vi "FT_Read_FT2232H_EEPROM.vi"(0 "Handle":u32) -> (1 "FT_Status":u32(ring) items=["FT_OK", "FT_INVALID_HANDLE", "FT_DEVICE_NOT_FOUND", "FT_DEVICE_NOT_OPENED", "FT_IO_ERROR", "FT_INSUFFICIENT_RESOURCES", "FT_INVALID_PARAMETER", "FT_INVALID_BAUD_RATE", "FT_DEVICE_NOT_OPENED_FOR_ERASE", "FT_DEVICE_NOT_OPENED_FOR_WRITE", "FT_FAILED_TO_WRITE_DEVICE", "FT_EEPROM_READ_FAILED", "FT_EEPROM_WRITE_FAILED", "FT_EEPROM_ERASE_FAILED", "FT_EEPROM_NOT_PRESENT", "FT_EEPROM_NOT_PROGRAMMED", "FT_INVALID_ARGS", "FT_NOT_SUPPORTED", "FT_OTHER_ERROR"], 2 "FT2232H EEPROM Contents":T1={"Vendor ID"=0, "Product ID"=0, "Manufacturer"="", "Manufacturer ID"="", "Description"="", "Serial Number"="", "Max Power (mA)"=0, "PnP"=0, "Self Powered"=0, "Remote Wake-Up"=0, "Pull Down Enable"=0, "Serial Number Enable 7"=0, "AL Slow Slew"=0, "AL Schmitt Input"=0, "AL Drive Current"=4, "AH Slow Slew"=0, "AH Schmitt Input"=0, "AH Drive Current"=4, "BL Slow Slew"=0, "BL Schmitt Input"=0, "BL Drive Current"=4, "BH Slow Slew"=0, "BH Schmitt Input"=0, "BH Drive Current"=4, "A Is 245 FIFO"=0, "A Is CPU FIFO"=0, "A Is Fast Serial"=0, "A Is VCP"=0, "B Is 245 FIFO"=0, "B Is CPU FIFO"=0, "B Is Fast Serial"=0, "B Is VCP"=0, "Power Save"=0} {"Power Save" items=["Disabled", "Enabled"]; "B Is VCP" items=["D2XX", "VCP"]; "B Is Fast Serial" items=["Disabled", "Enabled"]; "B Is CPU FIFO" items=["Disabled", "Enabled"]; "B Is 245 FIFO" items=["UART", "FIFO"]; "A Is VCP" items=["D2XX", "VCP"]; "A Is Fast Serial" items=["Disabled", "Enabled"]; "A Is CPU FIFO" items=["Disabled", "Enabled"]; "A Is 245 FIFO" items=["UART", "FIFO"]; "BH Drive Current" items=["4mA"=4, "8mA"=8, "12mA"=12, "16mA"=16]; "BH Schmitt Input" items=["Disabled", "Enabled"]; "BH Slow Slew" items=["Disabled", "Enabled"]; "BL Drive Current" items=["4mA"=4, "8mA"=8, "12mA"=12, "16mA"=16]; "BL Schmitt Input" items=["Disabled", "Enabled"]; "BL Slow Slew" items=["Disabled", "Enabled"]; "AH Drive Current" items=["4mA"=4, "8mA"=8, "12mA"=12, "16mA"=16]; "AH Schmitt Input" items=["Disabled", "Enabled"]; "AH Slow Slew" items=["Disabled", "Enabled"]; "AL Drive Current" items=["4mA"=4, "8mA"=8, "12mA"=12, "16mA"=16]; "AL Schmitt Input" items=["Disabled", "Enabled"]; "AL Slow Slew" items=["Disabled", "Enabled"]; "Serial Number Enable 7" items=["Disabled", "Enabled"]; "Pull Down Enable" items=["Disabled", "Enabled"]; "Remote Wake-Up" items=["Disabled", "Enabled"]; "Self Powered" items=["Bus Powered", "Self Powered"]; "PnP" items=["Disabled", "Enabled"]})   [LabVIEW 2019, in "D2XX_Functions.lvlib"]
uses:
  <userlib>/LevyLab/Relay Box/D2XX_Functions/D2XX_Functions.lvlib
  <userlib>/LevyLab/Relay Box/D2XX_Functions/i386/ftd2xx.dll
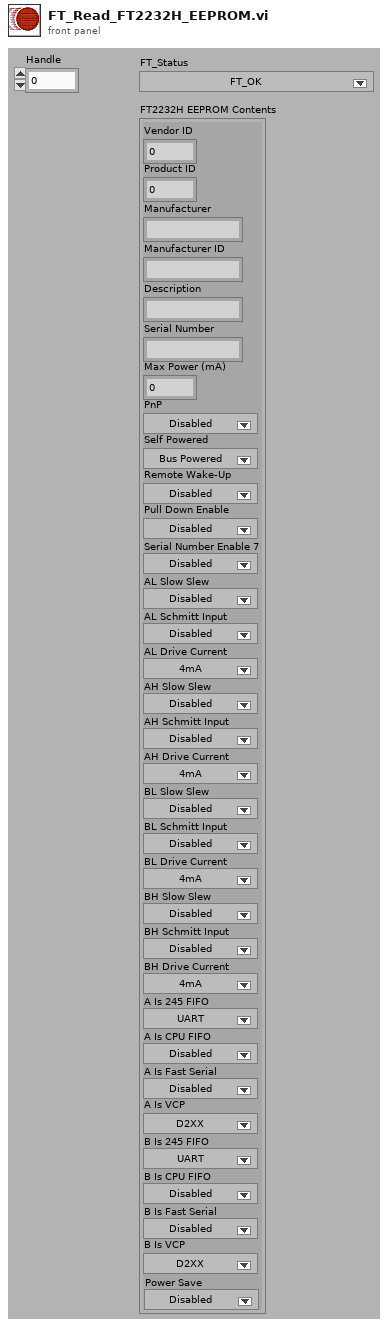
[diagram p1: front panel]
types:
  T1 = cluster{"Vendor ID":u16, "Product ID":u16, "Manufacturer":string, "Manufacturer ID":string, "Description":string, "Serial Number":string, "Max Power (mA)":u16, "PnP":u16, "Self Powered":u16, "Remote Wake-Up":u16, "Pull Down Enable":u8, "Serial Number Enable 7":u8, "AL Slow Slew":u8, "AL Schmitt Input":u8, "AL Drive Current":u8, "AH Slow Slew":u8, "AH Schmitt Input":u8, "AH Drive Current":u8, "BL Slow Slew":u8, "BL Schmitt Input":u8, "BL Drive Current":u8, "BH Slow Slew":u8, "BH Schmitt Input":u8, "BH Drive Current":u8, "A Is 245 FIFO":u8, "A Is CPU FIFO":u8, "A Is Fast Serial":u8, "A Is VCP":u8, "B Is 245 FIFO":u8, "B Is CPU FIFO":u8, "B Is Fast Serial":u8, "B Is VCP":u8, "Power Save":u8}
  T2 = cluster{"Signature 1":u32, "Signature 2":u32, "Version":u32, "Vendor ID":u16, "Product ID":u16, "Manufacturer":u32, "Manufacturer ID":u32, "Description":u32, "Serial Number":u32, "Max Power (mA)":u16, "PnP":u16, "Self Powered":u16, "Remote Wake-Up":u16, "Rev4":u8, "Iso In":u8, "Iso Out":u8, "Pull Down Enable":u8, "Serial Number Enable":u8, "USB Version Enable":u8, "USB Version":u16, "Rev5":u8, "Iso In A":u8, "Iso In B":u8, "Iso Out A":u8, "Iso Out B":u8, "Pull Down Enable 5":u8, "Serial Number Enable 5":u8, "USB Version Enable 5":u8, "USB Version 5":u16, "A Is High Current":u8, "B Is High Current":u8, "A Is 245 FIFO":u8, "A Is CPU FIFO":u8, "A Is Fast Serial":u8, "A Is VCP":u8, "B Is 245 FIFO":u8, "B Is CPU FIFO":u8, "B Is Fast Serial":u8, "B Is VCP":u8, "Use Ext Osc":u8, "High Drive IOs":u8, "Endpoint Size":u8, "Pull Down Enable R":u8, "Serial Number Enable R":u8, "Invert TXD":u8, "Invert RXD":u8, "Invert RTS":u8, "Invert CTS":u8, "Invert DTR":u8, "Invert DSR":u8, "Invert DCD":u8, "Invert RI":u8, "CBus0":u8, "CBus1":u8, "CBus2":u8, "CBus3":u8, "CBus4":u8, "R Is VCP":u8, "Pull Down Enable 7":u8, "Serial Number Enable 7":u8, "AL Slow Slew":u8, "AL Schmitt Input":u8, "AL Drive Current":u8, "AH Slow Slew":u8, "AH Schmitt Input":u8, "AH Drive Current":u8, "BL Slow Slew":u8, "BL Schmitt Input":u8, "BL Drive Current":u8, "BH Slow Slew":u8, "BH Schmitt Input":u8, "BH Drive Current":u8, "A Is 245 FIFO 7":u8, "A Is CPU FIFO 7":u8, "A Is Fast Serial 7":u8, "A Is VCP 7":u8, "B Is 245 FIFO 7":u8, "B Is CPU FIFO 7":u8, "B Is Fast Serial 7":u8, "B Is VCP 7":u8, "PowerSaveEnable":u8, "Pull Down Enable 8":u8, "Serial Number Enable 8":u8, "A Slow Slew":u8, "A Schmitt Input":u8, "A Drive Current":u8, "B Slow Slew":u8, "B Schmitt Input":u8, "B Drive Current":u8, "C Slow Slew":u8, "C Schmitt Input":u8, "C Drive Current":u8, "D Slow Slew":u8, "D Schmitt Input":u8, "D Drive Current":u8, "A RI Is TXDEN":u8, "B RI Is TXDEN":u8, "C RI Is TXDEN":u8, "D RI Is TXDEN":u8, "A Is VCP 8":u8, "B Is VCP 8":u8, "C Is VCP 8":u8, "D Is VCP 8":u8}
  T3 = cluster{"Vendor ID":u16, "Product ID":u16, "Manufacturer":string, "Manufacturer ID":string, "Description":string, "Serial Number":string, "Max Power (mA)":u16, "PnP":u16, "Self Powered":u16, "Remote Wake-Up":u16, "Pull Down Enable 7":u8, "Serial Number Enable 7":u8, "AL Slow Slew":u8, "AL Schmitt Input":u8, "AL Drive Current":u8, "AH Slow Slew":u8, "AH Schmitt Input":u8, "AH Drive Current":u8, "BL Slow Slew":u8, "BL Schmitt Input":u8, "BL Drive Current":u8, "BH Slow Slew":u8, "BH Schmitt Input":u8, "BH Drive Current":u8, "A Is 245 FIFO 7":u8, "A Is CPU FIFO 7":u8, "A Is Fast Serial 7":u8, "A Is VCP 7":u8, "B Is 245 FIFO 7":u8, "B Is CPU FIFO 7":u8, "B Is Fast Serial 7":u8, "B Is VCP 7":u8, "PowerSaveEnable":u8}
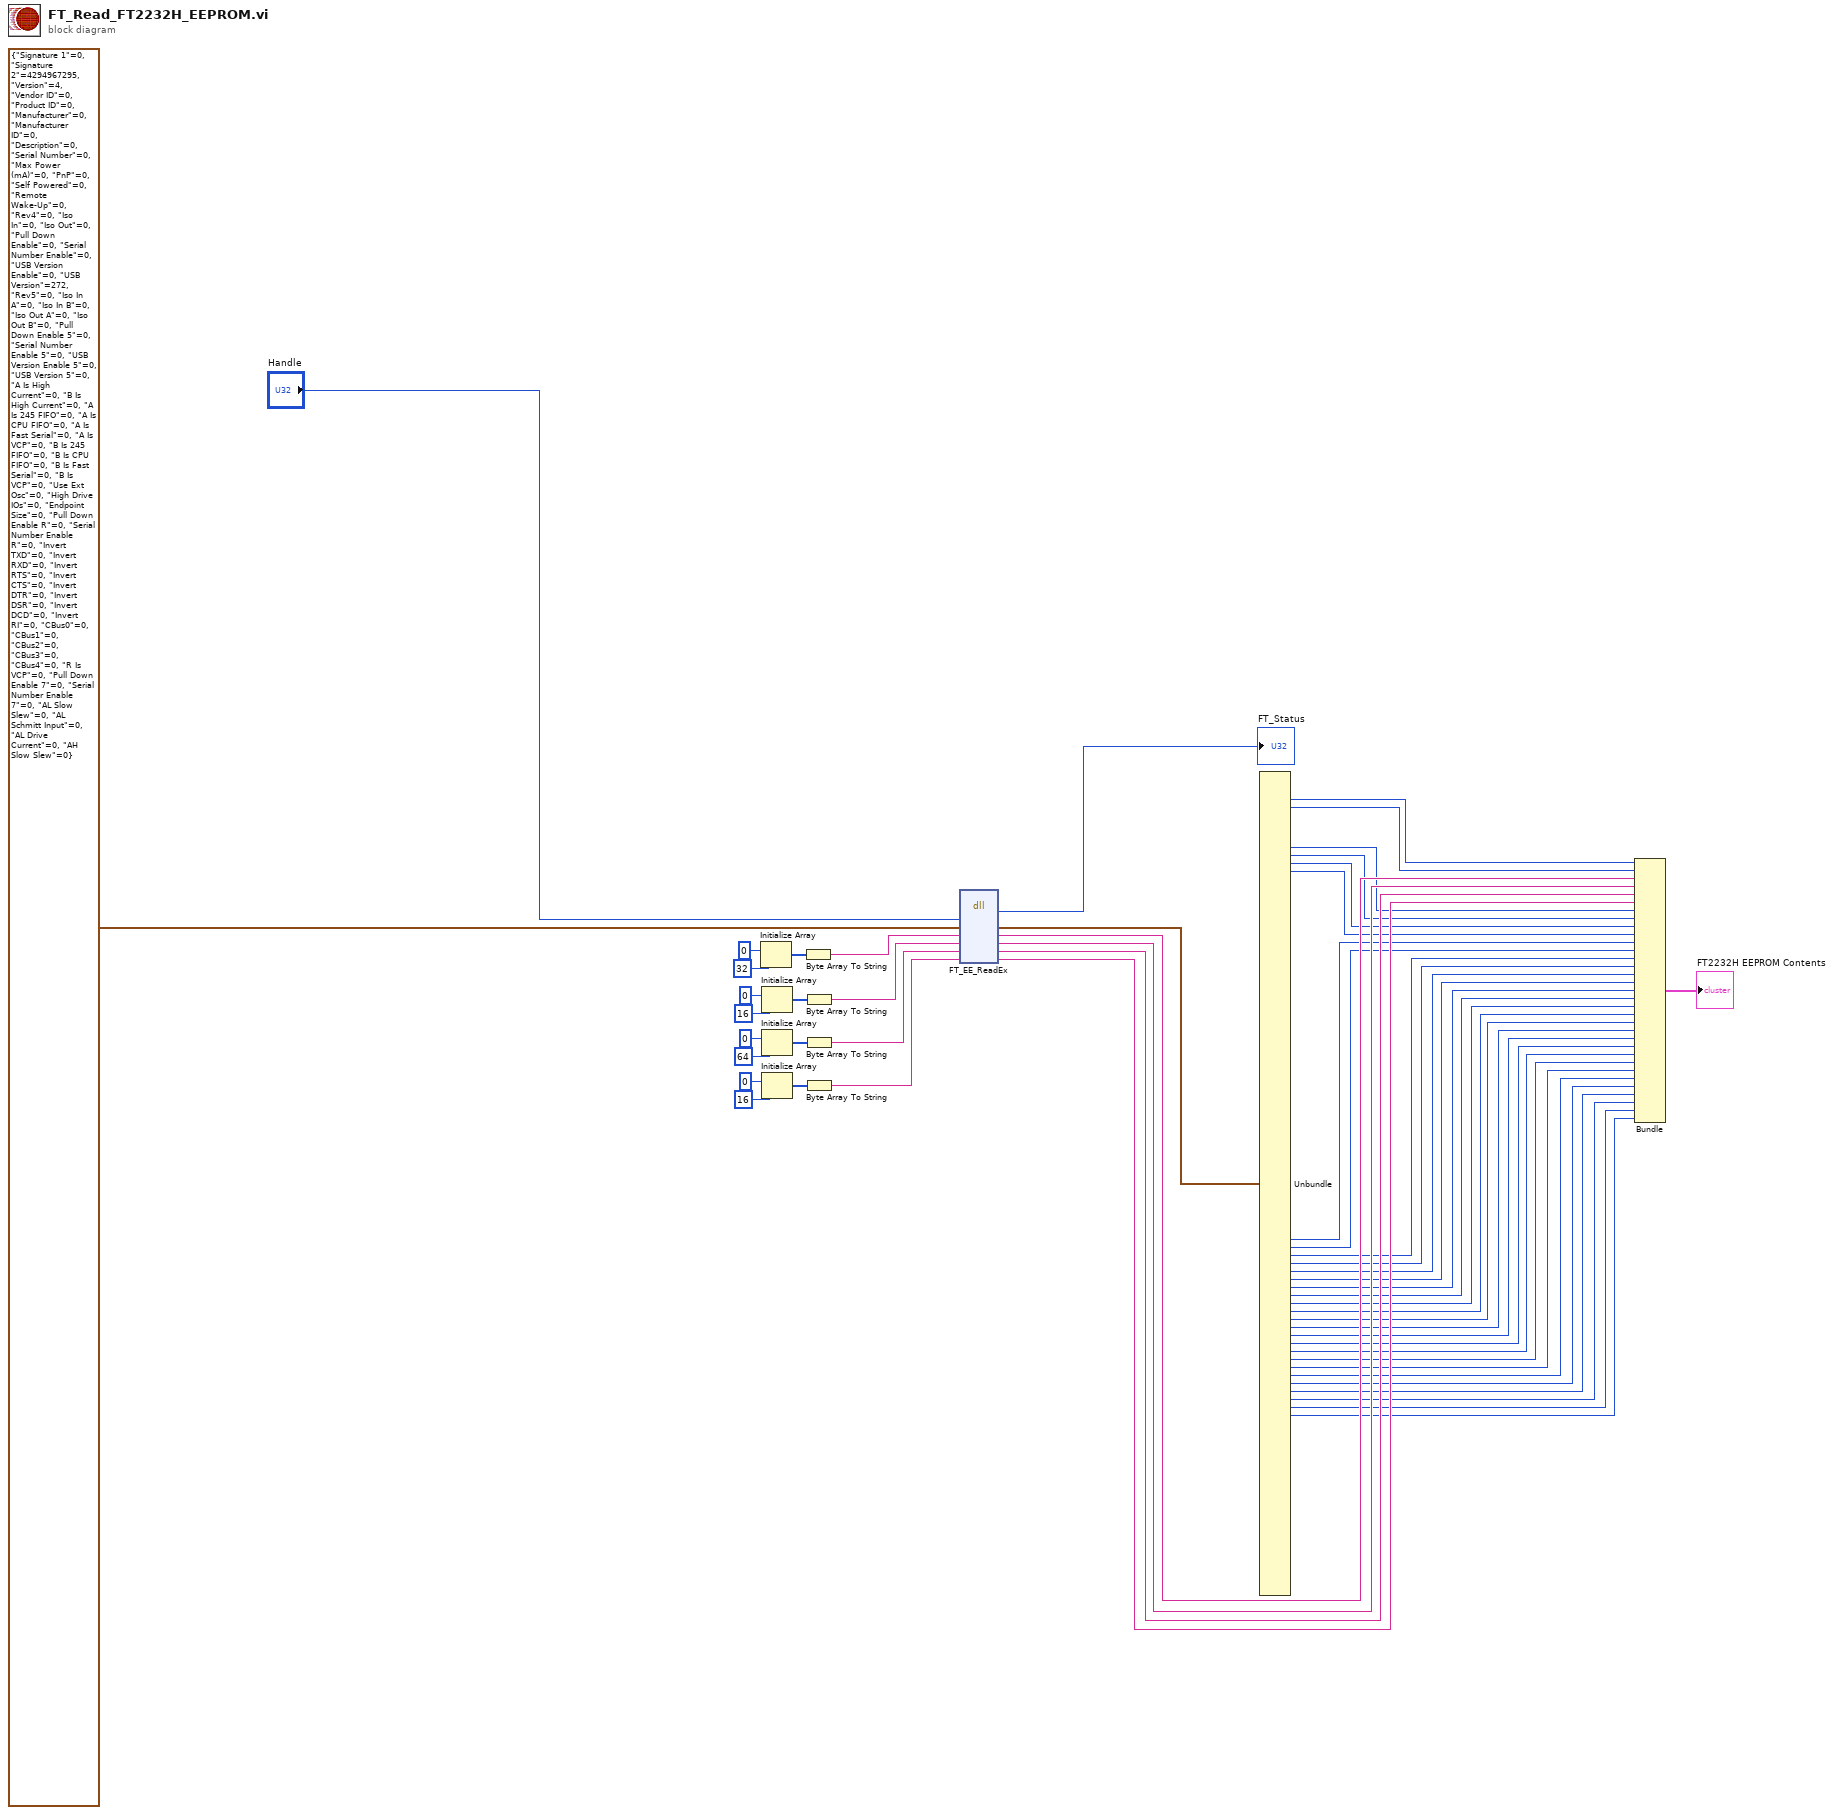
[diagram p0: block diagram]
diagram:
  n1 = Initialize Array(u8 0, 32 ("dimension size")) -> (w47:u8[])
  n2 = Initialize Array(u8 0, 16 ("dimension size")) -> (w45:u8[])
  n3 = Initialize Array(u8 0, 64 ("dimension size")) -> (w43:u8[])
  n4 = Initialize Array(u8 0, 16 ("dimension size")) -> (w41:u8[])
  n5 = Byte Array To String(unsigned byte array=w47) -> (string=w36:string)
  n6 = Byte Array To String(unsigned byte array=w45) -> (string=w35:string)
  n7 = Byte Array To String(unsigned byte array=w43) -> (string=w34:string)
  n8 = Byte Array To String(unsigned byte array=w41) -> (string=w33:string)
  n9 = dll-call lib="C:/Program Files (x86)/National Instruments/LabVIEW 2019/user.lib/LevyLab/Relay Box/D2XX_Functions/i386/FTD2XX.dll" fn="FT_EE_ReadEx"("Handle"="Handle", "FT232-FT245 EEPROM Contents 4"=T2 {"Signature 1"=0, "Signature 2"=4294967295, "Version"=4, "Vendor ID"=0, "Product ID"=0, "Manufacturer"=0, "Manufacturer ID"=0, "Description"=0, "Serial Number"=0, "Max Power (mA)"=0, "PnP"=0, "Self Powered"=0, "Remote Wake-Up"=0, "Rev4"=0, "Iso In"=0, "Iso Out"=0, "Pull Down Enable"=0, "Serial Number Enable"=0, "USB Version Enable"=0, "USB Version"=272, "Rev5"=0, "Iso In A"=0, "Iso In B"=0, "Iso Out A"=0, "Iso Out B"=0, "Pull Down Enable 5"=0, "Serial Number Enable 5"=0, "USB Version Enable 5"=0, "USB Version 5"=0, "A Is High Current"=0, "B Is High Current"=0, "A Is 245 FIFO"=0, "A Is CPU FIFO"=0, "A Is Fast Serial"=0, "A Is VCP"=0, "B Is 245 FIFO"=0, "B Is CPU FIFO"=0, "B Is Fast Serial"=0, "B Is VCP"=0, "Use Ext Osc"=0, "High Drive IOs"=0, "Endpoint Size"=0, "Pull Down Enable R"=0, "Serial Number Enable R"=0, "Invert TXD"=0, "Invert RXD"=0, "Invert RTS"=0, "Invert CTS"=0, "Invert DTR"=0, "Invert DSR"=0, "Invert DCD"=0, "Invert RI"=0, "CBus0"=0, "CBus1"=0, "CBus2"=0, "CBus3"=0, "CBus4"=0, "R Is VCP"=0, "Pull Down Enable 7"=0, "Serial Number Enable 7"=0, "AL Slow Slew"=0, "AL Schmitt Input"=0, "AL Drive Current"=0, "AH Slow Slew"=0, "AH Schmitt Input"=0, "AH Drive Current"=0, "BL Slow Slew"=0, "BL Schmitt Input"=0, "BL Drive Current"=0, "BH Slow Slew"=0, "BH Schmitt Input"=0, "BH Drive Current"=0, "A Is 245 FIFO 7"=0, "A Is CPU FIFO 7"=0, "A Is Fast Serial 7"=0, "A Is VCP 7"=0, "B Is 245 FIFO 7"=0, "B Is CPU FIFO 7"=0, "B Is Fast Serial 7"=0, "B Is VCP 7"=0, "PowerSaveEnable"=0, "Pull Down Enable 8"=0, "Serial Number Enable 8"=0, "A Slow Slew"=0, "A Schmitt Input"=0, "A Drive Current"=0, "B Slow Slew"=0, "B Schmitt Input"=0, "B Drive Current"=0, "C Slow Slew"=0, "C Schmitt Input"=0, "C Drive Current"=0, "D Slow Slew"=0, "D Schmitt Input"=0, "D Drive Current"=0, "A RI Is TXDEN"=0, "B RI Is TXDEN"=0, "C RI Is TXDEN"=0, "D RI Is TXDEN"=0, "A Is VCP 8"=0, "B Is VCP 8"=0, "C Is VCP 8"=0, "D Is VCP 8"=0}, "Manufacturer"=w36, "Manufacturer ID"=w35, "Description"=w34, "Serial Number"=w33) -> ("FT_Status"=→"FT_Status":u32, "FT232-FT245 EEPROM Contents 4"=w31:T2, "Manufacturer"=w50:string, "Manufacturer ID"=w52:string, "Description"=w51:string, "Serial Number"=w49:string)  [unwired: 4 in, 2 out]
  n10 = Unbundle(w31) -> ("Vendor ID"=w30:u16, "Product ID"=w29:u16, "Max Power (mA)"=w28:u16, "PnP"=w27:u16, "Self Powered"=w26:u16, "Remote Wake-Up"=w25:u16, "Pull Down Enable 7"=w24:u8, "Serial Number Enable 7"=w23:u8, "AL Slow Slew"=w22:u8, "AL Schmitt Input"=w21:u8, "AL Drive Current"=w20:u8, "AH Slow Slew"=w19:u8, "AH Schmitt Input"=w18:u8, "AH Drive Current"=w17:u8, "BL Slow Slew"=w16:u8, "BL Schmitt Input"=w15:u8, "BL Drive Current"=w14:u8, "BH Slow Slew"=w13:u8, "BH Schmitt Input"=w12:u8, "BH Drive Current"=w11:u8, "A Is 245 FIFO 7"=w10:u8, "A Is CPU FIFO 7"=w9:u8, "A Is Fast Serial 7"=w8:u8, "A Is VCP 7"=w7:u8, "B Is 245 FIFO 7"=w6:u8, "B Is CPU FIFO 7"=w5:u8, "B Is Fast Serial 7"=w4:u8, "B Is VCP 7"=w3:u8, "PowerSaveEnable"=w2:u8)  [unwired: 74 out]
  n11 = Bundle("Vendor ID"=w30, "Product ID"=w29, "Manufacturer"=w50, "Manufacturer ID"=w52, "Description"=w51, "Serial Number"=w49, "Max Power (mA)"=w28, "PnP"=w27, "Self Powered"=w26, "Remote Wake-Up"=w25, "Pull Down Enable 7"=w24, "Serial Number Enable 7"=w23, "AL Slow Slew"=w22, "AL Schmitt Input"=w21, "AL Drive Current"=w20, "AH Slow Slew"=w19, "AH Schmitt Input"=w18, "AH Drive Current"=w17, "BL Slow Slew"=w16, "BL Schmitt Input"=w15, "BL Drive Current"=w14, "BH Slow Slew"=w13, "BH Schmitt Input"=w12, "BH Drive Current"=w11, "A Is 245 FIFO 7"=w10, "A Is CPU FIFO 7"=w9, "A Is Fast Serial 7"=w8, "A Is VCP 7"=w7, "B Is 245 FIFO 7"=w6, "B Is CPU FIFO 7"=w5, "B Is Fast Serial 7"=w4, "B Is VCP 7"=w3, "PowerSaveEnable"=w2) -> (→"FT2232H EEPROM Contents":T3)  [unwired: 1 in]
